vi "CRY6181.vi"() -> ()   [LabVIEW 2013]
doc: "This VI is an adaptation of a splash screen VI developed by Steve Harrision for \"Serving Up Powerful Solutions: LabVIEW VI Server Examples\" - an article which originally appeared in the LabVIEW Technical Resource newsletter, Vol. 6 Number 4. In this example, the diagram has been simplified by replacing the original text status with a progress bar. Refer to the diagram notes and accompanying text for more details.\n\nSubscribe to the LabVIEW Technical Resource newsletter! LTR is a quarterly publication providing technical information to LabVIEW system developers.\n\nFor subscription information, back issues, and LTR VI Code Paks contact:\nLTR Publishing, Inc. \n6060 N. Central Expressway, Suite 502\nDallas, TX 75206\n(214) 706-0587\nFAX (214) 706-0506\nE-mail: subscribe@ltrpub.com\nwww.ltrpub.com"
uses:
  CRYMainGlobal.vi
  CRYWindow/SubVI/CRYMain Sub Window Global.vi
panel:
  out "Minimized":bool
  out "Hidden":bool
  out "Message Copyright":string
  out "Message HomePage":string
  out "Message Version":string
  out "Message String":string
  out "Chinese":bool
  out "English":bool
  out "Korean":bool
  out "error out 2":errorcluster
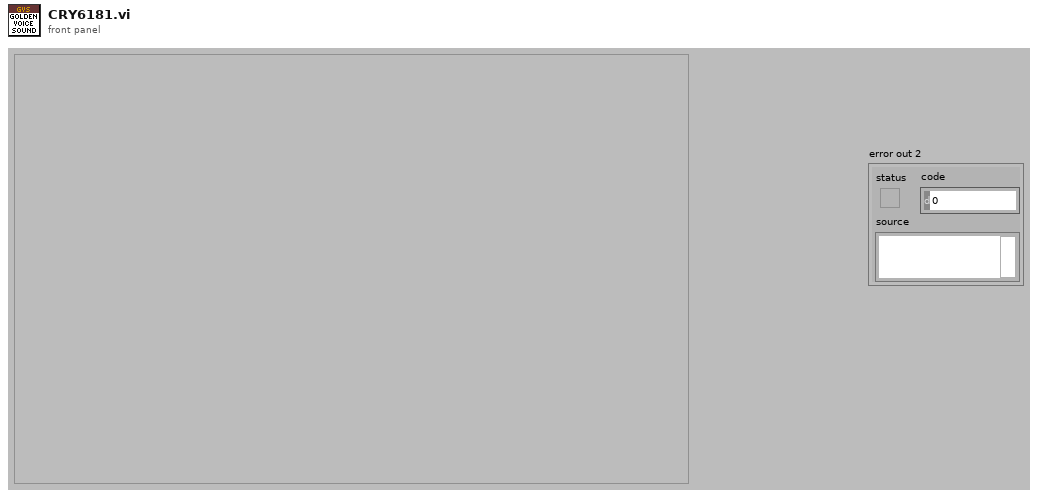
[diagram p1: front panel]
types:
  T1 = enum32{"English", "Chinese", "Korean", "Japanese", "Russian", "Chinese traditional"}
  T2 = enum32{"Invalid", "Standard", "Closed", "Hidden", "Minimized", "Maximized"}
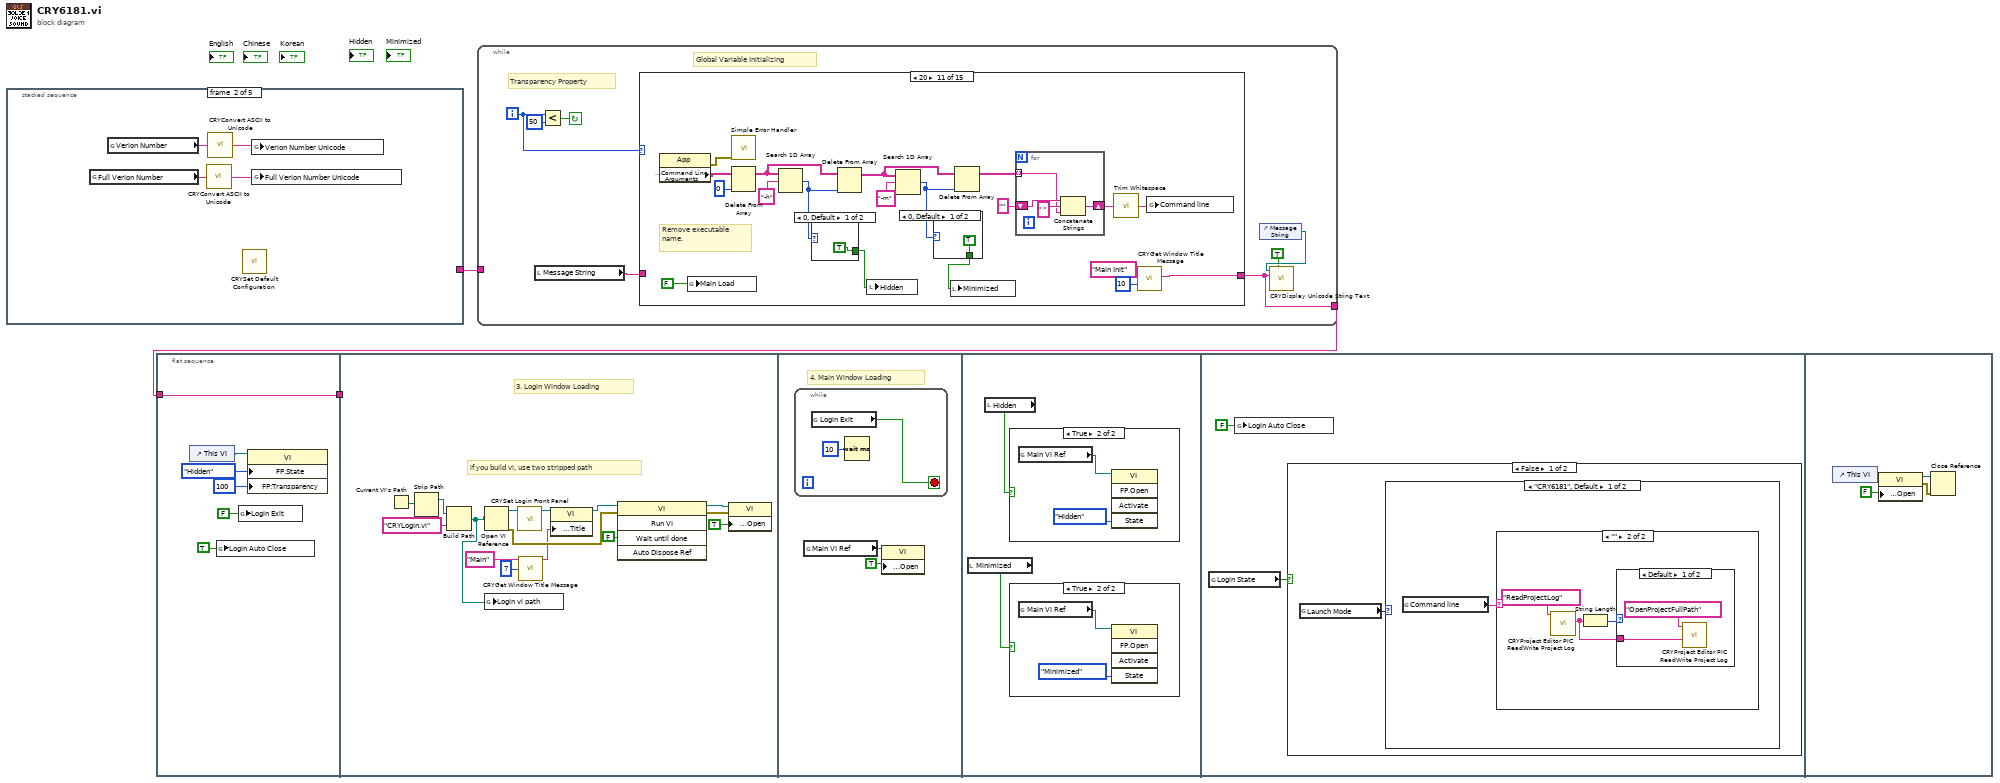
[diagram p0: block diagram]
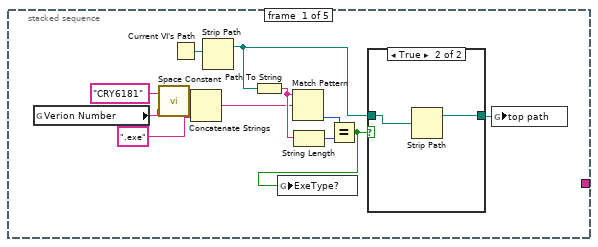
[diagram p2: hidden frame]
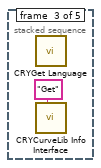
[diagram p4: hidden frame]
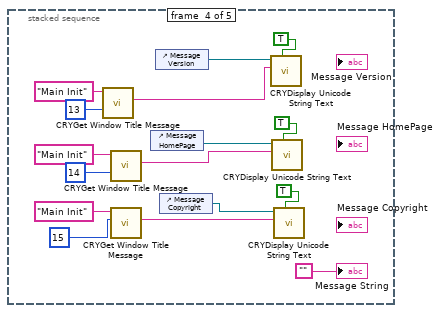
[diagram p5: hidden frame]
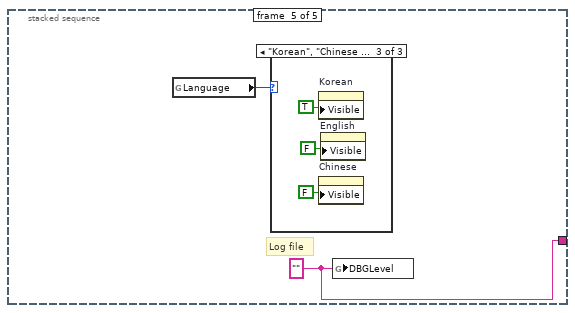
[diagram p6: hidden frame]
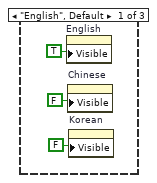
[diagram p7: hidden frame]
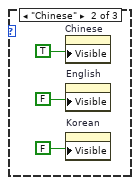
[diagram p8: hidden frame]
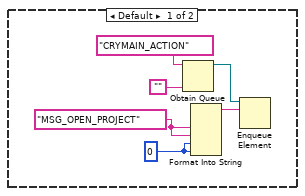
[diagram p11: hidden frame]
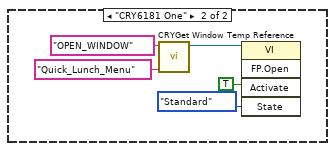
[diagram p13: hidden frame]
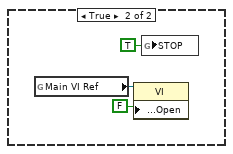
[diagram p14: hidden frame]
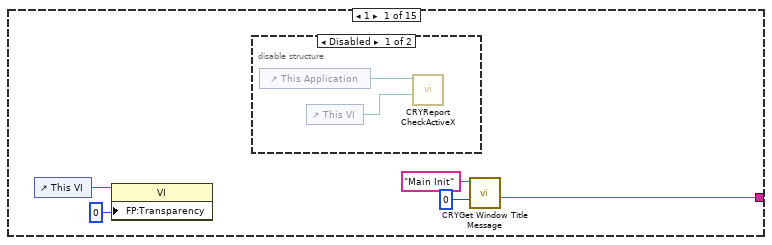
[diagram p15: hidden frame]
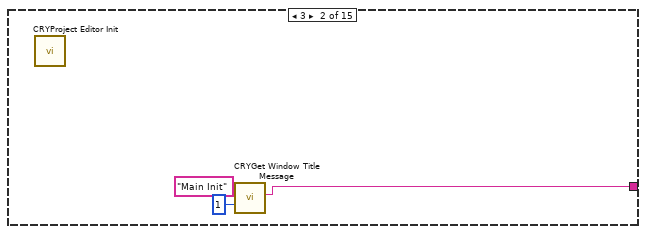
[diagram p17: hidden frame]
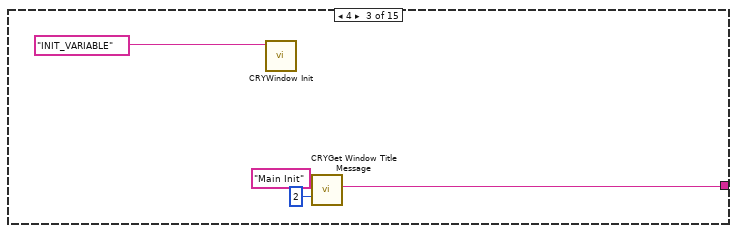
[diagram p18: hidden frame]
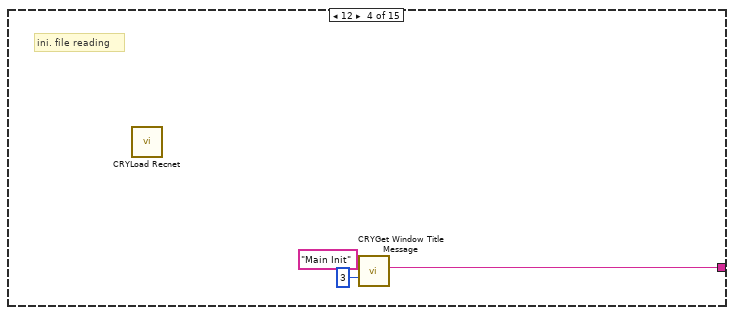
[diagram p19: hidden frame]
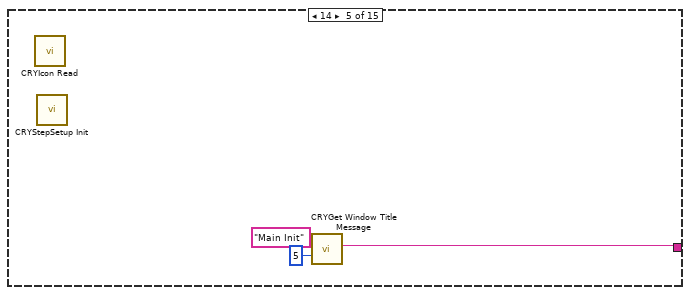
[diagram p20: hidden frame]
diagram:
  n1 = stacked-sequence {
    tunnel: [_ _ _ _ w40] -> w1
    frame #0 {
      n2 = global read "CRYMainGlobal.vi" "Verion Number"() -> (w6:string)
      n3 = call <vilib>:"Space Constant.vi"() -> ("String"=w7:string)
      n4 = Current VI's Path() -> (path=w9:path)
      n5 = Concatenate Strings("CRY6181" ("ini file name"), w7, w6, ".exe" ("ini file name")) -> (w4:string)
      n6 = Strip Path(path=w9) -> (stripped path=w13:path)  [unwired: 1 out]
      n7 = Path To String(path=w13) -> (string=w12:string)
      n8 = Match Pattern(string=w12, regular expression=w4) -> (offset past match=w10:i32)  [unwired: 4 out]
      n9 = String Length(string=w12) -> (length=w11:i32)
      n10 = Equal?(x=w10, y=w11) -> (x = y?=w15:bool)
      n11 = global write "CRYMainGlobal.vi" "ExeType?"(w15) -> ()
      n12 = case shown="True" w15 {
        tunnel: w13 -> [w16 w18]
        tunnel: [w16 w17] -> w14
        frame False {
        }
        frame True {
          n13 = Strip Path(path=w18) -> (stripped path=w17:path)  [unwired: 1 out]
        }
      }
      n14 = global write "CRYMainGlobal.vi" "top path"(w14) -> ()
    }
    frame #1 {
      n15 = global read "CRYMainGlobal.vi" "Full Verion Number"() -> (w21:string)
      n16 = global read "CRYMainGlobal.vi" "Verion Number"() -> (w22:string)
      n17 = call "CRYConvert ASCII to Unicode.vi"("ASCII"=w21) -> ("Unicode"=w19:string)  [unwired: 4 in]
      n18 = call "CRYConvert ASCII to Unicode.vi"("ASCII"=w22) -> ("Unicode"=w20:string)  [unwired: 4 in]
      n19 = call "CRYSet Default Configuration.vi"() -> ()  [unwired: 3 out]
      n20 = global write "CRYMainGlobal.vi" "Verion Number Unicode"(w20) -> ()
      n21 = global write "CRYMainGlobal.vi" "Full Verion Number Unicode"(w19) -> ()
    }
    frame #2 {
      n22 = call "CRYGet Language.vi"() -> ()  [unwired: 12 in]
      n23 = call "CRYCurveLib Info Interface.vi"("sAction"="Get") -> ()  [unwired: 11 in]
    }
    frame #3 {
      n24 = call "CRYGet Window Title Message.vi"("No"=13, "Kind"="Main Init") -> ("Unicode String"=w32:string)  [unwired: 4 in, 5 out]
      n25 = call "CRYGet Window Title Message.vi"("No"=14, "Kind"="Main Init") -> ("Unicode String"=w26:string)  [unwired: 4 in, 5 out]
      n26 = call "CRYGet Window Title Message.vi"("No"=15, "Kind"="Main Init") -> ("Unicode String"=w28:string)  [unwired: 4 in, 5 out]
      n27 = control-ref of="Message HomePage"() -> (w25:refnum<vi>)
      n28 = control-ref of="Message Version"() -> (w31:refnum<vi>)
      n29 = control-ref of="Message Copyright"() -> (w29:refnum<vi>)
      n30 = call "CRYDisplay Unicode String Text.vi"("Interpret as Unicode (T)"=TRUE, "String Value"=w32, "String Control Reference"=w31) -> ()  [unwired: 5 in, 2 out]
      n31 = call "CRYDisplay Unicode String Text.vi"("Interpret as Unicode (T)"=TRUE, "String Value"=w26, "String Control Reference"=w25) -> ()  [unwired: 5 in, 2 out]
      n32 = call "CRYDisplay Unicode String Text.vi"("Interpret as Unicode (T)"=TRUE, "String Value"=w28, "String Control Reference"=w29) -> ()  [unwired: 5 in, 2 out]
      "Message String" <- "" ("Message String")
    }
    frame #4 {
      w40 = "" ("DBGLevel")
      # "Log file"
      n33 = global read "CRYMainGlobal.vi" "Language"() -> (w41:T1)
      n34 = case shown="\"Korean\", \"Chinese traditional\"" w41 {
        frame "English", Default {
          n35 = property on="English" class="Bool (strict)"("Visible"=TRUE) -> ()  [unwired: 2 in, 2 out]
          n36 = property on="Chinese" class="Bool (strict)"("Visible"=FALSE) -> ()  [unwired: 2 in, 2 out]
          n37 = property on="Korean" class="Bool (strict)"("Visible"=FALSE) -> ()  [unwired: 2 in, 2 out]
        }
        frame "Chinese" {
          n38 = property on="Chinese" class="Bool (strict)"("Visible"=TRUE) -> ()  [unwired: 2 in, 2 out]
          n39 = property on="English" class="Bool (strict)"("Visible"=FALSE) -> ()  [unwired: 2 in, 2 out]
          n40 = property on="Korean" class="Bool (strict)"("Visible"=FALSE) -> ()  [unwired: 2 in, 2 out]
        }
        frame "Korean", "Chinese traditional" {
          n41 = property on="Korean" class="Bool (strict)"("Visible"=TRUE) -> ()  [unwired: 2 in, 2 out]
          n42 = property on="Chinese" class="Bool (strict)"("Visible"=FALSE) -> ()  [unwired: 2 in, 2 out]
          n43 = property on="English" class="Bool (strict)"("Visible"=FALSE) -> ()  [unwired: 2 in, 2 out]
        }
      }
      n44 = global write "CRYMain Sub Window Global.vi" "DBGLevel"(w40) -> ()
    }
  }
  n45 = flat-sequence {
    tunnel: w2 -> [w56]
    tunnel: [w56] -> w3
    tunnel: w3 -> [_]
    frame #0 {
      n46 = control-ref of="This VI"() -> (w54:refnum<vi>)
      n47 = global write "CRYMainGlobal.vi" "Login Auto Close"(TRUE ("Login Auto Close")) -> ()
      n48 = global write "CRYMainGlobal.vi" "Login Exit"(FALSE ("Login Exit")) -> ()
      n49 = property class="VI"(reference=w54, "FP.State"=T2."Hidden" ("Front Panel Window:State"), "FP:Transparency"=u8 100 ("Front Panel Window:Transparency")) -> ()  [unwired: 1 in, 2 out]
    }
    frame #1 {
      # "if you build vi, use two stripped path"
      # "3. Login Window Loading"
      n50 = Current VI's Path() -> (path=w66:path)
      n51 = Strip Path(path=w66) -> (stripped path=w65:path)  [unwired: 1 out]
      n52 = Build Path(base path=w65, name or relative path="CRYLogin.vi") -> (appended path=w57:path)
      n53 = Open VI Reference(vi path=w57) -> (vi reference=w64:refnum<vi>, error out=w69:errorcluster)  [unwired: 1 in, 4 out]
      n54 = global write "CRYMainGlobal.vi" "Login vi path"(w57) -> ()
      n55 = call "CRYSet Login Front Panel.vi"("Vi Ref in"=w64) -> ("Vi Ref out"=w60:refnum<vi>)  [unwired: 10 in]
      n56 = call "CRYGet Window Title Message.vi"("No"=7, "Kind"="Main") -> ("Multibyte String"=w61:string)  [unwired: 4 in, 5 out]
      n57 = property class="VI"(reference=w60, "Front Panel.Title"=w61) -> (reference out=w59:refnum<vi>)  [unwired: 1 in, 1 out]
      n58 = invoke class="VI" method="Run VI"(reference=w59, error in=w69, "Wait until done"=FALSE) -> (reference out=w68:refnum<vi>, error out=w67:errorcluster)  [unwired: 2 in, 3 out]
      n59 = property class="VI"(reference=w68, error in=w67, "Front Panel Window:Open"=TRUE ("Front Panel.Open")) -> ()  [unwired: 2 out]
    }
    frame #2 {
      # "4. Main Window Loading"
      n60 = while {
        stop <- w75 stop-if-true
        n61 = global read "CRYMainGlobal.vi" "Login Exit"() -> (w75:bool)
        n62 = Wait (ms)(milliseconds to wait=u32 10) -> ()  [unwired: 1 out]
      }
      n63 = global read "CRYMain Sub Window Global.vi" "Main VI Ref"() -> (w73:refnum<vi>)
      n64 = property class="VI"(reference=w73, "Front Panel Window:Open"=TRUE ("Front Panel.Open")) -> ()  [unwired: 1 in, 2 out]
    }
    frame #3 {
      n65 = local read "Minimized"() -> (w76:bool)
      n66 = local read "Hidden"() -> (w77:bool)
      n67 = case shown="True" w77 {
        frame False {
        }
        frame True {
          n68 = global read "CRYMain Sub Window Global.vi" "Main VI Ref"() -> (w81:refnum<vi>)
          n69 = invoke class="VI" method="FP.Open"(reference=w81, "State"=T2."Hidden") -> ()  [unwired: 3 in, 5 out]
        }
      }
      n70 = case shown="True" w76 {
        frame False {
        }
        frame True {
          n71 = global read "CRYMain Sub Window Global.vi" "Main VI Ref"() -> (w79:refnum<vi>)
          n72 = invoke class="VI" method="FP.Open"(reference=w79, "State"=T2."Minimized") -> ()  [unwired: 3 in, 5 out]
        }
      }
    }
    frame #4 {
      n73 = global read "CRYMainGlobal.vi" "Login State"() -> (w83:bool)
      n74 = global write "CRYMainGlobal.vi" "Login Auto Close"(FALSE ("Login Auto Close")) -> ()
      n75 = case shown="False" w83 {
        frame False {
          n76 = global read "CRYMainGlobal.vi" "Launch Mode"() -> (w84:enum32{"CRY6181", "CRY6181 One"})
          n77 = case shown="\"CRY6181\", Default" w84 {
            frame "CRY6181", Default {
              n78 = global read "CRYMainGlobal.vi" "Command line"() -> (w85:string)
              n79 = case shown="\"\"" w85 {
                frame Default {
                  w86 = 0 ("input 3")
                  w91 = "MSG_OPEN_PROJECT" ("input 1")
                  n80 = Obtain Queue(name (unnamed)="CRYMAIN_ACTION" ("YAxisTitle"), element data type="" ("Action Type")) -> (queue out=w90:refnum<queue>)  [unwired: 3 in, 2 out]
                  n81 = Format Into String(w91, w91, w86, w86) -> (resulting string=w89:string)  [unwired: 3 in, 1 out]
                  n82 = Enqueue Element(queue=w90, element=w89) -> ()  [unwired: 1 in, 4 out]
                }
                frame "" {
                  n83 = call "CRYProject Editor PIC ReadWrite Project Log.vi"("sAction"="ReadProjectLog") -> ("sData_Out"=w92:string)  [unwired: 9 in, 1 out]
                  n84 = String Length(string=w92) -> (length=w93:i32)
                  n85 = case shown="Default" w93 {
                    tunnel: w92 -> [w95 _]
                    frame Default {
                      n86 = call "CRYProject Editor PIC ReadWrite Project Log.vi"("sData"=w95, "sAction"="OpenProjectFullPath") -> ()  [unwired: 8 in, 2 out]
                    }
                    frame 0 {
                    }
                  }
                }
              }
            }
            frame "CRY6181 One" {
              n87 = call "CRYGet Window Temp Reference.vi"("sWindowName"="Quick_Lunch_Menu", "sAction"="OPEN_WINDOW") -> ("pVIRef_Out"=w97:refnum<vi>)  [unwired: 5 in, 4 out]
              n88 = invoke class="VI" method="FP.Open"(reference=w97, "Activate"=TRUE ("Activate?"), "State"=T2."Standard") -> ()  [unwired: 2 in, 5 out]
            }
          }
        }
        frame True {
          n89 = global read "CRYMain Sub Window Global.vi" "Main VI Ref"() -> (w102:refnum<vi>)
          n90 = property class="VI"(reference=w102, "Front Panel Window:Open"=FALSE ("Front Panel.Open")) -> ()  [unwired: 1 in, 2 out]
          n91 = global write "CRYMainGlobal.vi" "STOP"(TRUE ("STOP")) -> ()
        }
      }
    }
    frame #5 {
      n92 = control-ref of="This VI"() -> (w105:refnum<vi>)
      n93 = property class="VI"(reference=w105, "Front Panel.Open"=FALSE ("Front Panel Window:Open")) -> (reference out=w107:refnum<vi>, error out=w106:errorcluster)  [unwired: 1 in]
      n94 = Close Reference(reference=w107, error in (no error)=w106) -> ()  [unwired: 1 out]
    }
  }
  n95 = while {
    tunnel: [w112] -> w2
    tunnel: w1 -> [_]
    i -> [w114]
    stop <- w115 continue-if-true
    # "Global Variable Initializing"
    # "Transparency Property"
    n96 = local read "Message String"() -> (w113:string)
    n97 = Less?(x=w114, y=50) -> (x < y?=w115:bool)
    n98 = case shown="20" w114 {
      tunnel: [w118 w123 w126 w130 w133 w136 w139 w143 w146 w150 w165 w186 w193 "" w206] -> w112
      tunnel: w113 -> [_ _ _ _ _ _ _ _ _ _ _ w186 w193 _ w206]
      frame 1 {
        n99 = control-ref of="This VI"() -> (w117:refnum<vi>)
        n100 = property class="VI"(reference=w117, "FP:Transparency"=u8 0 ("Front Panel Window:Transparency")) -> ()  [unwired: 1 in, 2 out]
        n101 = disable-structure shown="Disabled" {
          frame Disabled {
            n102 = control-ref of="This Application"() -> (w121:refnum<vi>)
            n103 = control-ref of="This VI"() -> (w122:refnum<vi>)
            n104 = call "CRYReport CheckActiveX.vi"("pVIRef"=w122, "pApplication"=w121) -> ()  [unwired: 10 in]
          }
          frame Enabled {
          }
        }
        n105 = call "CRYGet Window Title Message.vi"("No"=0, "Kind"="Main Init") -> ("Unicode String"=w118:string)  [unwired: 4 in, 5 out]
      }
      frame 3 {
        n106 = call "CRYProject Editor Init.vi"() -> ()  [unwired: 12 out]
        n107 = call "CRYGet Window Title Message.vi"("No"=1, "Kind"="Main Init") -> ("Unicode String"=w123:string)  [unwired: 4 in, 5 out]
      }
      frame 4 {
        n108 = call "CRYWindow Init.vi"("sAction"="INIT_VARIABLE") -> ()  [unwired: 11 in]
        n109 = call "CRYGet Window Title Message.vi"("No"=2, "Kind"="Main Init") -> ("Unicode String"=w126:string)  [unwired: 4 in, 5 out]
      }
      frame 12 {
        # "ini. file reading"
        n110 = call "CRYLoad Recnet.vi"() -> ()  [unwired: 2 in, 1 out]
        n111 = call "CRYGet Window Title Message.vi"("No"=3, "Kind"="Main Init") -> ("Unicode String"=w130:string)  [unwired: 4 in, 5 out]
      }
      frame 14 {
        n112 = call "CRYIcon Read.vi"() -> ()  [unwired: 9 in, 1 out]
        n113 = call "CRYStepSetup Init.vi"() -> ()  [unwired: 12 in]
        n114 = call "CRYGet Window Title Message.vi"("No"=5, "Kind"="Main Init") -> ("Unicode String"=w133:string)  [unwired: 4 in, 5 out]
      }
      frame 15 {
        n115 = call "CRYInit Curve Library.vi"() -> ()  [unwired: 1 out]
        n116 = call "CRYGet Window Title Message.vi"("No"=4, "Kind"="Main Init") -> ("Unicode String"=w136:string)  [unwired: 4 in, 5 out]
      }
      frame 16 {
        n117 = call "CRYStep Contents Init.vi"() -> ()  [unwired: 12 out]
        n118 = call "CRYGet Window Title Message.vi"("No"=6, "Kind"="Main Init") -> ("Unicode String"=w139:string)  [unwired: 4 in, 5 out]
      }
      frame 17 {
        w142 = u8 0 ("Port 1 Pattern")
        # "Digital IO initialization"
        n119 = call "CRYMessage Set DigitalIO Ports.vi"("Port 2 Pattern"=w142, "Port 1 Pattern"=w142) -> ()  [unwired: 7 in, 3 out]
        n120 = call "CRYGet Window Title Message.vi"("No"=7, "Kind"="Main Init") -> ("Unicode String"=w143:string)  [unwired: 4 in, 5 out]
      }
      frame 18 {
        n121 = call "CRYLoad Virtual Data.vi"() -> ("error out"=→"error out 2":errorcluster)  [unwired: 1 in, 10 out]
        n122 = call "CRYGet Window Title Message.vi"("No"=8, "Kind"="Main Init") -> ("Unicode String"=w146:string)  [unwired: 4 in, 5 out]
      }
      frame 19 {
        n123 = call "CRYOperator Process.vi"("sAction"="Init Data") -> ()  [unwired: 10 in, 1 out]
        n124 = call "CRYGet Window Title Message.vi"("No"=9, "Kind"="Main Init") -> ("Unicode String"=w150:string)  [unwired: 4 in, 5 out]
      }
      frame 20 {
        # "Remove executable\nname."
        n125 = property class="App"() -> (error out=w171:errorcluster, "Application:Command Line Arguments"=w169:string[])  [unwired: 2 in, 1 out]
        n126 = global write "CRYMainGlobal.vi" "Main Load"(FALSE ("Main Load")) -> ()
        n127 = call <vilib>:"Simple Error Handler.vi"("error in (no error)"=w171) -> ()  [unwired: 1 in, 8 out]
        n128 = Delete From Array(array=w169, index=0 ("length")) -> (array with subset deleted=w161:string[])  [unwired: 1 in, 1 out]
        n129 = Search 1D Array(1D array=w161, element="-h") -> (index of element=w157:i32)  [unwired: 1 in]
        n130 = case shown="0, Default" w157 {
          tunnel: [TRUE ("Hidden") FALSE ("Hidden")] -> w155
          frame 0, Default {
          }
          frame -1 {
          }
        }
        n131 = Delete From Array(array=w161, index=w157) -> (array with subset deleted=w159:string[])  [unwired: 1 in, 1 out]
        n132 = local write "Hidden"(w155) -> ()
        n133 = Search 1D Array(1D array=w159, element="-m") -> (index of element=w156:i32)  [unwired: 1 in]
        n134 = case shown="0, Default" w156 {
          tunnel: [TRUE ("Hidden") FALSE ("Hidden")] -> w154
          frame 0, Default {
          }
          frame -1 {
          }
        }
        n135 = local write "Minimized"(w154) -> ()
        n136 = Delete From Array(array=w159, index=w156) -> (array with subset deleted=w158:string[])  [unwired: 1 in, 1 out]
        n137 = for {
          tunnel: w158 -> [w177] mode=indexing
          shift-right: [w179] -> w168
          shift-left: "" -> [w180]
          n138 = Concatenate Strings(w180, " " ("string"), w177) -> (w179:string)
        }
        n139 = call <vilib>:"Trim Whitespace.vi"("string"=w168) -> ("trimmed string"=w163:string)  [unwired: 1 in]
        n140 = call "CRYGet Window Title Message.vi"("No"=10, "Kind"="Main Init") -> ("Unicode String"=w165:string)  [unwired: 4 in, 5 out]
        n141 = global write "CRYMainGlobal.vi" "Command line"(w163) -> ()
      }
      frame 21 {
        # "4. Login Widow Loading"
        n142 = Current VI's Path() -> (path=w185:path)
        n143 = Strip Path(path=w185) -> (stripped path=w181:path)  [unwired: 1 out]
        n144 = Build Path(base path=w181, name or relative path="CRYMain.vi") -> (appended path=w182:path)
        n145 = Open VI Reference(vi path=w182) -> (vi reference=w184:refnum<vi>)  [unwired: 1 in, 5 out]
        n146 = disable-structure shown="Disabled" {
          disable-tunnel: w184 -> [w192 _]
          frame Disabled {
            n147 = call "CRYLoad Main Configure.vi"("vi reference in"=w192) -> ()  [unwired: 1 in, 2 out]
          }
          frame Enabled {
          }
        }
        n148 = property class="VI"(reference=w184, "Front Panel Window:Open"=FALSE ("Front Panel.Open")) -> (reference out=w189:refnum<vi>, error out=w188:errorcluster)  [unwired: 1 in]
        n149 = call "CRYSet TooBar and StatusBar.vi"("Type"="Init Toolbar", "MainVI Ref In"=w184) -> ()  [unwired: 2 in, 8 out]
        n150 = invoke class="VI" method="Run VI"(reference=w189, error in=w188, "Wait until done"=FALSE) -> ()  [unwired: 2 in, 5 out]
      }
      frame 22 {
        n151 = while {
          i -> [w199]
          stop <- w204 stop-if-true
          n152 = global read "CRYMainGlobal.vi" "Main Load"() -> (w204:bool)
          n153 = Quotient & Remainder(x=w199, y=3) -> (x-y*floor(x/y)=w197:i32)  [unwired: 1 out]
          n154 = Add(x=10 ("No"), y=w197) -> (x+y=w198:i32)
          n155 = control-ref of="Message String"() -> (w196:refnum<vi>)
          n156 = call "CRYGet Window Title Message.vi"("No"=w198, "Kind"="Main Init") -> ("Unicode String"=w194:string)  [unwired: 4 in, 5 out]
          n157 = call "CRYDisplay Unicode String Text.vi"("Interpret as Unicode (T)"=TRUE, "String Value"=w194, "String Control Reference"=w196) -> ()  [unwired: 5 in, 2 out]
          n158 = Wait (ms)(milliseconds to wait=u32 150) -> ()  [unwired: 1 out]
        }
      }
      frame 49 {
      }
      frame Default {
      }
    }
    n159 = control-ref of="Message String"() -> (w111:refnum<vi>)
    n160 = call "CRYDisplay Unicode String Text.vi"("Interpret as Unicode (T)"=TRUE, "String Value"=w112, "String Control Reference"=w111) -> ()  [unwired: 5 in, 2 out]
  }
